vi "Motor de Passo LabView.vi"() -> ()   [LabVIEW 2010]
uses:
  <vilib>/LabVIEW Interface for Arduino/Type Defs/Pin Mode.ctl
  <vilib>/LabVIEW Interface for Arduino/LabVIEW Interface for Arduino.lvlib
  <userlib>/NI_Timer/NI_Timer.lvlib
panel:
  in  "Microseconds 2":dbl
  in  "Microseconds":dbl
  in  "stop":bool
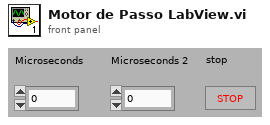
[diagram p1: front panel]
types:
  T1 = typedef "LabVIEW Interface for Arduino.lvlib/Pin Mode.ctl" = enum8{"Input", "Output"}
  T2 = typedef "LabVIEW Interface for Arduino.lvlib/Arduino Resource.ctl" = cluster{"VISA resource":refnum<visa-resource-name>, "Board Type":T3, "Connection Type":enum8{"USB / Serial"}, "Bytes Per Packet (15)":u8}
  T3 = typedef "LabVIEW Interface for Arduino.lvlib/Board Type.ctl" = enum16{"Uno", "Dimuelanove w/Atmega 328", "Mega 2560"}
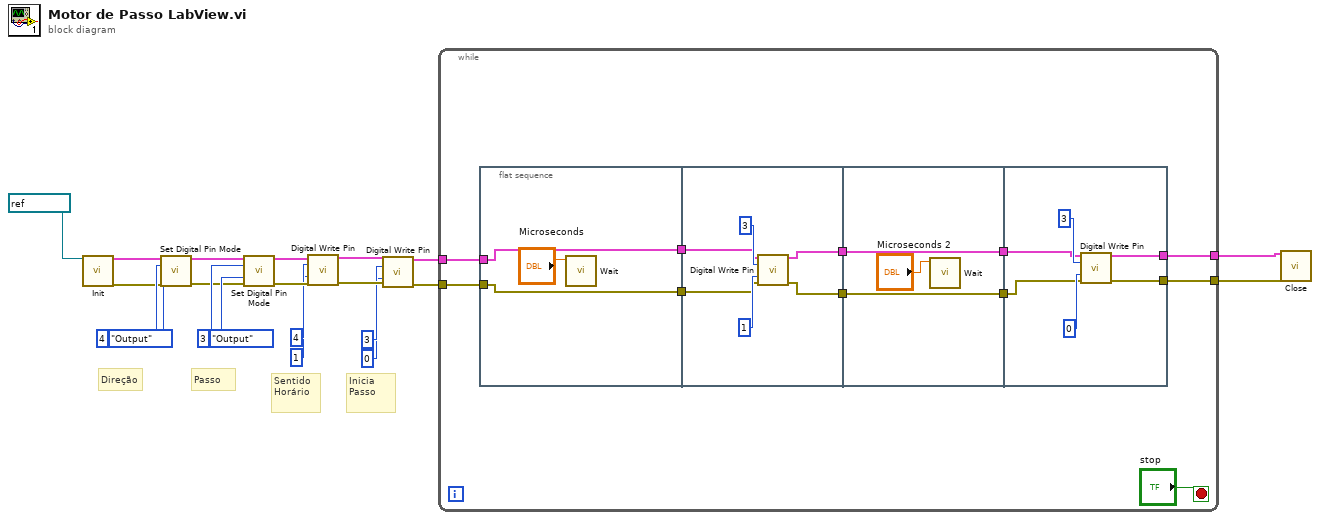
[diagram p0: block diagram]
diagram:
  # "Inicia Passo"
  # "Sentido Horário"
  # "Passo"
  # "Direção"
  n1 = call <vilib>:"Init.vi"("VISA resource"=refnum<visa-resource-name> "COM4") -> ("Arduino Resource"=w20:T2, "error out"=w14:errorcluster)  [unwired: 17 in]
  n2 = call <vilib>:"Set Digital Pin Mode.vi"("Arduino Resource"=w20, "Digital I/O Pin"=u8 4, "Pin Mode (Input)"=Pin_Mode."Output", "error in"=w14) -> ("Arduino Resource"=w19:T2, "error out"=w13:errorcluster)  [unwired: 10 in]
  n3 = call <vilib>:"Set Digital Pin Mode.vi"("Arduino Resource"=w19, "Digital I/O Pin"=u8 3, "Pin Mode (Input)"=Pin_Mode."Output", "error in"=w13) -> ("Arduino Resource"=w10:T2, "error out"=w9:errorcluster)  [unwired: 10 in]
  n4 = call <vilib>:"Digital Write Pin.vi"("Arduino Resource"=w10, "Digital I/O Pin (0)"=u8 4, "Value (0)"=u8 1, "error in"=w9) -> ("Arduino Resource"=w12:T2, "error out"=w11:errorcluster)  [unwired: 10 in]
  n5 = call <vilib>:"Digital Write Pin.vi"("Arduino Resource"=w12, "Digital I/O Pin (0)"=u8 3, "Value (0)"=u8 0, "error in"=w11) -> ("Arduino Resource"=w4:T2, "error out"=w3:errorcluster)  [unwired: 10 in]
  n6 = while {
    tunnel: w4 -> [w26]
    tunnel: w3 -> [w25]
    tunnel: [w23] -> w2
    tunnel: [w22] -> w1
    stop <- "stop" stop-if-true
    n7 = flat-sequence {
      tunnel: w26 -> [w35]
      tunnel: w25 -> [w34]
      tunnel: [w35] -> w32
      tunnel: [w34] -> w31
      tunnel: w32 -> [w39]
      tunnel: w31 -> [w38]
      tunnel: [w37] -> w30
      tunnel: [w36] -> w29
      tunnel: w30 -> [w44]
      tunnel: [w44] -> w28
      tunnel: w29 -> [w43]
      tunnel: [w43] -> w27
      tunnel: w28 -> [w48]
      tunnel: w27 -> [w47]
      tunnel: [w46] -> w23
      tunnel: [w45] -> w22
      frame #0 {
        n8 = call <userlib>:"Wait.vi"("delay"="Microseconds") -> ()  [unwired: 11 in]
      }
      frame #1 {
        n9 = call <vilib>:"Digital Write Pin.vi"("Arduino Resource"=w39, "Digital I/O Pin (0)"=u8 3, "Value (0)"=u8 1, "error in"=w38) -> ("Arduino Resource"=w37:T2, "error out"=w36:errorcluster)  [unwired: 10 in]
      }
      frame #2 {
        n10 = call <userlib>:"Wait.vi"("delay"="Microseconds 2") -> ()  [unwired: 11 in]
      }
      frame #3 {
        n11 = call <vilib>:"Digital Write Pin.vi"("Arduino Resource"=w48, "Digital I/O Pin (0)"=u8 3, "Value (0)"=u8 0, "error in"=w47) -> ("Arduino Resource"=w46:T2, "error out"=w45:errorcluster)  [unwired: 10 in]
      }
    }
  }
  n12 = call <vilib>:"Close.vi"("Arduino Resource"=w2, "error in"=w1) -> ()  [unwired: 13 in, 1 out]
